vi "Format Markdown Table.vi"(8 "Error In":errorcluster, 10 "Unformatted Header Cluster":T1, 11 "Unformatted Numeric Array":dbl[][](array[numeric])) -> (0 "Error Out":errorcluster, 3 "Formatted Array to Markdown Table":string)   [LabVIEW 2017]
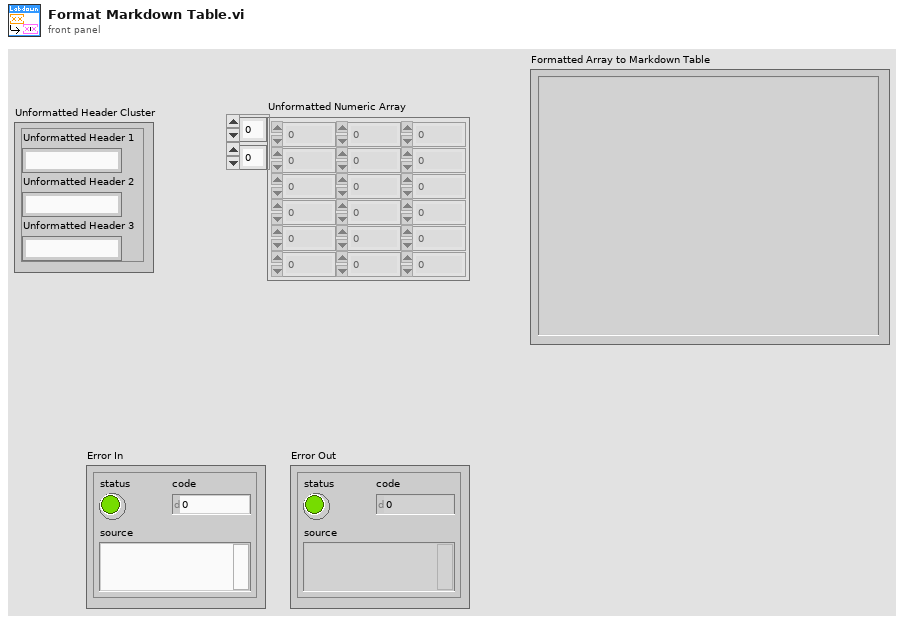
[diagram p1: front panel]
types:
  T1 = cluster{"Unformatted Header 1":string, "Unformatted Header 2":string, "Unformatted Header 3":string}
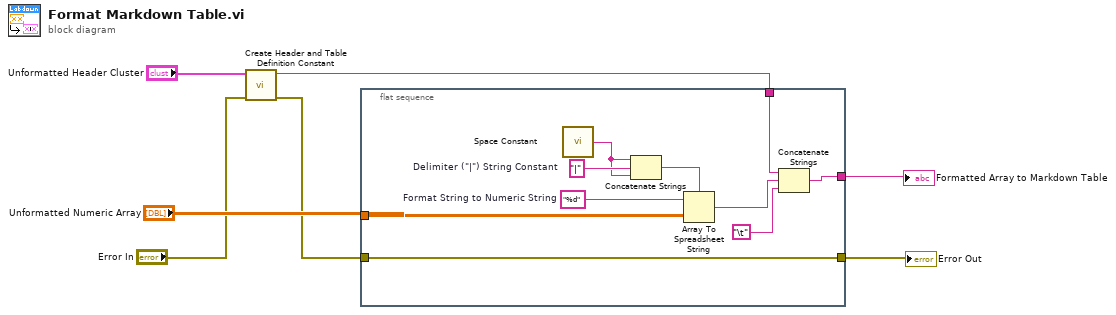
[diagram p0: block diagram]
diagram:
  n1 = call "Create Header and Table Definition Constant.vi"("Error In"="Error In", "Header Cluster"="Unformatted Header Cluster") -> ("Error Out"=w4:errorcluster, "Output Header and Table Constant"=w2:string)  [unwired: 8 in]
  n2 = flat-sequence {
    tunnel: "Unformatted Numeric Array" -> [w16]
    tunnel: w4 -> [w15]
    tunnel: [w15] -> w6
    tunnel: w2 -> [w12]
    tunnel: [w10] -> w1
    frame #0 {
      w13 = "|"  # Delimiter ("|") String Constant
      w17 = "%d"  # Format String to Numeric String
      n3 = call <vilib>:"Space Constant.vi"() -> ("String"=w9:string)
      n4 = Concatenate Strings(w9, w13, w9) -> (w14:string)
      n5 = Array To Spreadsheet String(delimiter (Tab)=w14, array=w16, 3:w17) -> (spreadsheet string=w11:string)
      n6 = Concatenate Strings(w12, w11, "\t") -> (w10:string)
    }
  }
  "Formatted Array to Markdown Table" <- w1
  "Error Out" <- w6
